vi "K2450 Set Volt.vi"(8 "error in (no error)":errorcluster {"code" format="%.0x"}, 10 "Voltage 2450":dbl, 11 "VISA resource name":refnum<visa-resource-name>) -> (0 "error out":errorcluster {"code" format="%.0x"}, 3 "dup VISA Session":refnum<visa-resource-name>)   [LabVIEW 2019]
panel:
  # "Make sure unit is set to source V\nsour:func volt\nAnd turned on\nOUTPut ON"
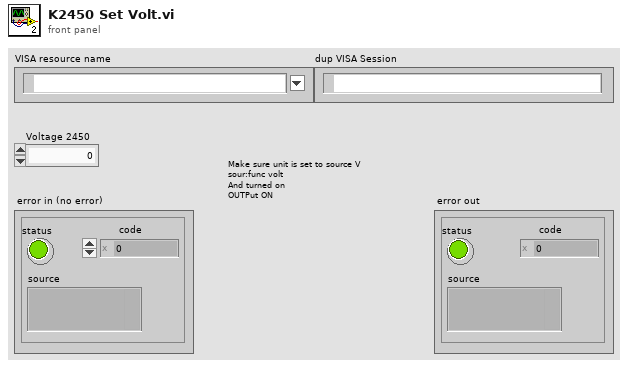
[diagram p1: front panel]
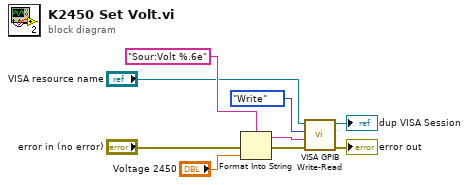
[diagram p0: block diagram]
diagram:
  n1 = Format Into String(format string="Sour:Volt %.6e" ("Command"), error in="error in (no error)", "Voltage 2450") -> (resulting string=w5:string, error out=w3:errorcluster)  [unwired: 1 in]
  n2 = call "VISA GPIB Write-Read.vi"("error in (no error)"=w3, "Command"=w5, "Action"=enum16{"Write", "Read", "Write & Read"}."Write", "VISA resource name"="VISA resource name") -> ("error out"=→"error out":errorcluster, "dup VISA Session"=→"dup VISA Session":refnum<visa-resource-name>)  [unwired: 4 in, 2 out]
